vi "Transfer Group.Set Debug Flags.vi"(10 "Debug Flags":refnum<class "DSF.Engine.Debug Flags.lvclass">, 11 "Transfer Group in":refnum<class "Transfer Group.lvclass">) -> (3 "Transfer Group out":refnum<class "Transfer Group.lvclass">)   [LabVIEW 2017, in "DSF.Engine.lvlib" / "Transfer Group.lvclass"]
uses:
  Transfer Group.lvclass
  Debug/DSF.Engine.Debug Flags.lvclass
  Transfer Group.lvclass/Transfer Group.ctl
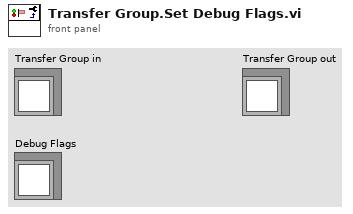
[diagram p1: front panel]
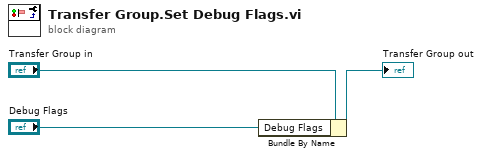
[diagram p0: block diagram]
diagram:
  n1 = Bundle By Name(cluster="Transfer Group in", "Debug Flags"="Debug Flags") -> (→"Transfer Group out":refnum<class "Transfer Group.lvclass">)
